vi "deadzone_sharp.vi"(1 "Size":dbl, 2 "in":dbl) -> (0 "out":dbl)   [LabVIEW 2023]
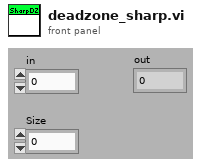
[diagram p1: front panel]
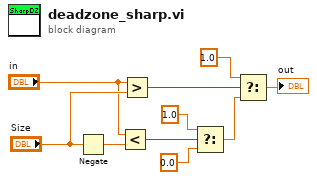
[diagram p0: block diagram]
diagram:
  n1 = Negate(x="Size") -> (-x=w5:dbl)
  n2 = Less?(x="in", y=w5) -> (x < y?=w3:bool)
  n3 = Greater?(x="in", y="Size") -> (0:w9:bool)
  n4 = Select(t=1.0, s=w3, f=0.0) -> (s? t:f=w7:dbl)
  n5 = Select(t=1.0, s=w9, f=w7) -> (s? t:f=→"out":dbl)
